vi "Speed_Read(SPD).vi"(4 "baud rate (9600)":u32=115200 caption="보 전송속도(9600)", 5 "Port":refnum<visa-resource-name>="COM4" caption="VISA 리소스 이름") -> (0 "Speed(Y)":i32, 1 "Speed(X)":i32, 2 "Read Buffer":string)   [LabVIEW 2016]
uses:
  <vilib>/Instr/_visa.llb/VISA Flush IO Buffer Mask.ctl
  <vilib>/Instr/_visa.llb/VISA Configure Serial Port (Instr).vi
panel:
  out "에러 출력":errorcluster
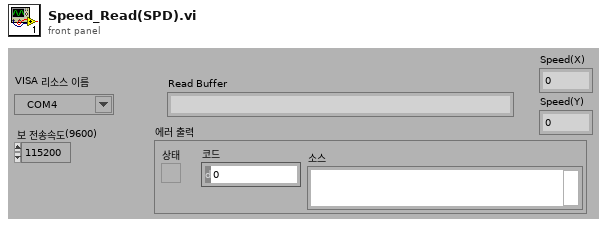
[diagram p1: front panel]
types:
  T1 = typedef "VISA Flush IO Buffer Mask.ctl" = u16
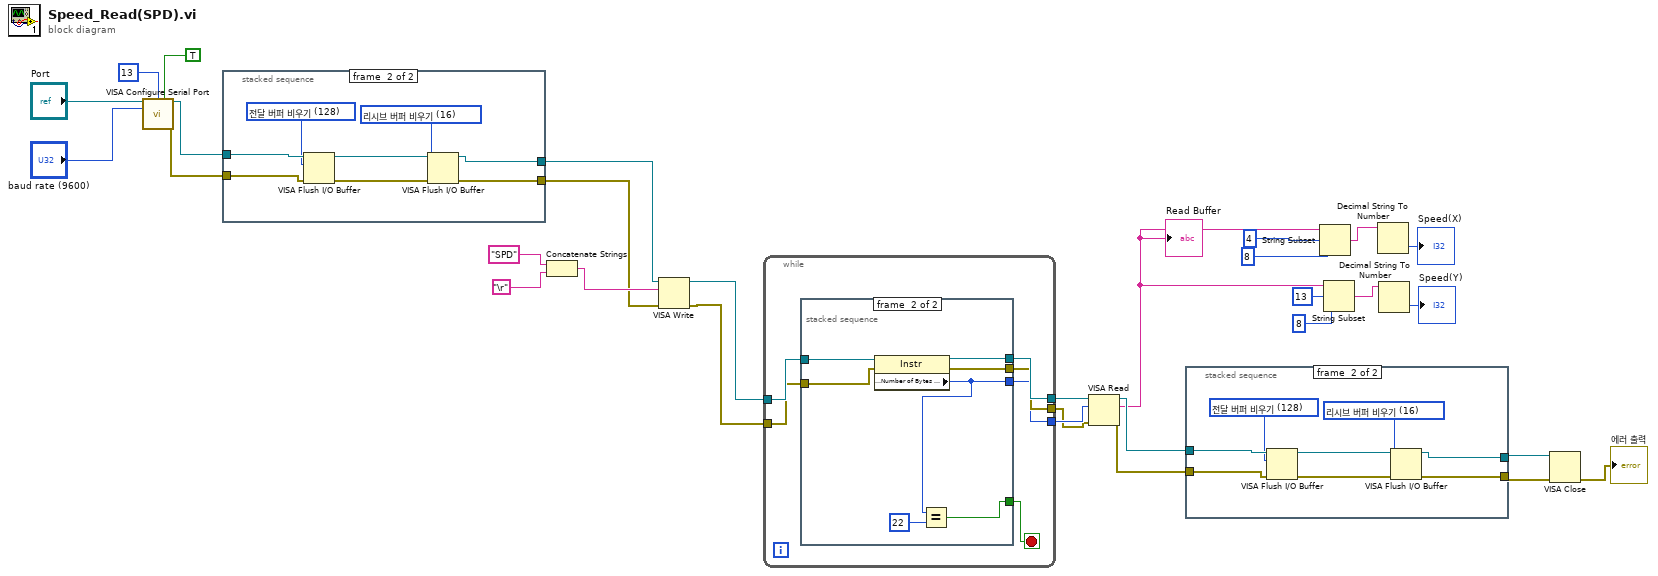
[diagram p0: block diagram]
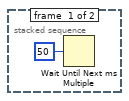
[diagram p2: hidden frame]
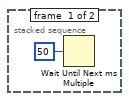
[diagram p3: hidden frame]
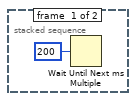
[diagram p4: hidden frame]
diagram:
  n1 = call-poly "VISA Configure Serial Port"("VISA resource name"="Port", "termination char\n(0xA = '\\n' = LF)"=i16 13 ("termination char\n(0xA = '\\n' = LF)"), "Enable Termination\nChar (T)"=TRUE ("Enable Termination\nChar (T)"), "baud rate (9600)"="baud rate (9600)") -> ("VISA resource name out"=w13:refnum<visa-resource-name>, "error out"=w12:errorcluster)  [unwired: 10 in]
  n2 = stacked-sequence {
    tunnel: w13 -> [_ w39]
    tunnel: w12 -> [_ w38]
    tunnel: [_ w34] -> w11
    tunnel: [_ w33] -> w10
    frame #0 {
      n3 = Wait Until Next ms Multiple(millisecond multiple=u32 50 ("ms 배수")) -> ()  [unwired: 1 out]
    }
    frame #1 {
      w32 = T1 16 items=["리시브 버퍼 비우기"=16, "전달 버퍼 디바이스에 쓰기"=32, "리시브 버퍼 비우기(I/O 없음)"=64, "전달 버퍼 비우기"=128] ("Mask")
      w37 = T1 128 items=["리시브 버퍼 비우기"=16, "전달 버퍼 디바이스에 쓰기"=32, "리시브 버퍼 비우기(I/O 없음)"=64, "전달 버퍼 비우기"=128] ("Mask")
      n4 = VISA Flush I/O Buffer(VISA resource name=w39, mask (16)=w37, error in (no error)=w38) -> (VISA resource name out=w36:refnum<visa-resource-name>, error out=w35:errorcluster)
      n5 = VISA Flush I/O Buffer(VISA resource name=w36, mask (16)=w32, error in (no error)=w35) -> (VISA resource name out=w34:refnum<visa-resource-name>, error out=w33:errorcluster)
    }
  }
  n6 = Concatenate Strings("SPD" ("버퍼 쓰기"), "\r") -> (w27:string)
  n7 = VISA Write(VISA resource name=w11, write buffer=w27, error in (no error)=w10) -> (VISA resource name out=w25:refnum<visa-resource-name>, error out=w24:errorcluster)  [unwired: 1 out]
  n8 = while {
    tunnel: w25 -> [w45]
    tunnel: w24 -> [w44]
    tunnel: [w43] -> w26
    tunnel: [w40] -> w19
    tunnel: [w42] -> w18
    stop <- w41 stop-if-true
    n9 = stacked-sequence {
      tunnel: w45 -> [_ w53]
      tunnel: w44 -> [_ w52]
      tunnel: [_ w51] -> w43
      tunnel: [_ w50] -> w42
      tunnel: [_ w48] -> w41
      tunnel: [_ w47] -> w40
      frame #0 {
        n10 = Wait Until Next ms Multiple(millisecond multiple=u32 200 ("ms 배수")) -> ()  [unwired: 1 out]
      }
      frame #1 {
        n11 = property class="Instr"(reference=w53, error in=w52) -> (reference out=w51:refnum<visa-resource-name>, error out=w50:errorcluster, "Serial Settings:Number of Bytes at Serial Port"=w47:u32)
        n12 = Equal?(x=w47, y=u32 22) -> (x = y?=w48:bool)
      }
    }
  }
  n13 = VISA Read(VISA resource name=w26, byte count=w19, error in (no error)=w18) -> (VISA resource name out=w23:refnum<visa-resource-name>, read buffer=w9:string, error out=w22:errorcluster)  [unwired: 1 out]
  "Read Buffer" <- w9
  n14 = stacked-sequence {
    tunnel: w23 -> [_ w62]
    tunnel: w22 -> [_ w61]
    tunnel: [_ w57] -> w21
    tunnel: [_ w56] -> w20
    frame #0 {
      n15 = Wait Until Next ms Multiple(millisecond multiple=u32 50 ("ms 배수")) -> ()  [unwired: 1 out]
    }
    frame #1 {
      w55 = T1 16 items=["리시브 버퍼 비우기"=16, "전달 버퍼 디바이스에 쓰기"=32, "리시브 버퍼 비우기(I/O 없음)"=64, "전달 버퍼 비우기"=128] ("Mask")
      w60 = T1 128 items=["리시브 버퍼 비우기"=16, "전달 버퍼 디바이스에 쓰기"=32, "리시브 버퍼 비우기(I/O 없음)"=64, "전달 버퍼 비우기"=128] ("Mask")
      n16 = VISA Flush I/O Buffer(VISA resource name=w62, mask (16)=w60, error in (no error)=w61) -> (VISA resource name out=w59:refnum<visa-resource-name>, error out=w58:errorcluster)
      n17 = VISA Flush I/O Buffer(VISA resource name=w59, mask (16)=w55, error in (no error)=w58) -> (VISA resource name out=w57:refnum<visa-resource-name>, error out=w56:errorcluster)
    }
  }
  n18 = String Subset(string=w9, offset (0)=4 ("오프셋(0)"), length (rest)=8 ("길이(나머지)")) -> (substring=w4:string)
  n19 = String Subset(string=w9, offset (0)=13 ("오프셋(0)"), length (rest)=8 ("길이(나머지)")) -> (substring=w3:string)
  n20 = Decimal String To Number(string=w4) -> (number=→"Speed(X)":i32)  [unwired: 2 in, 1 out]
  n21 = Decimal String To Number(string=w3) -> (number=→"Speed(Y)":i32)  [unwired: 2 in, 1 out]
  n22 = VISA Close(VISA resource name=w21, error in (no error)=w20) -> (error out=→"에러 출력":errorcluster)
